vi "Write Sine Grap to binary file.vi"() -> ()   [LabVIEW 2020]
uses:
  <vilib>/Analysis/NI_AALBase.lvlib
panel:
  in  "Path":path
  out "Array":dbl[](array[numeric])
  out "Waveform Graph":dbl[](graph)
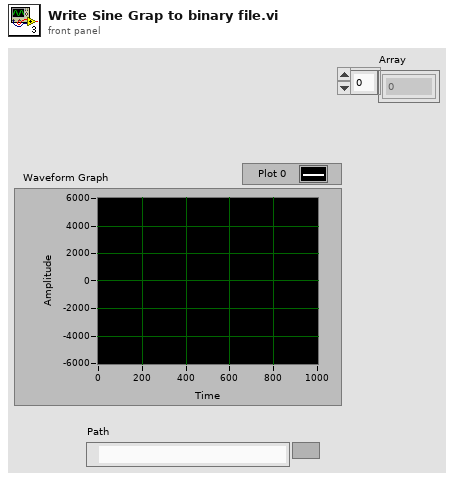
[diagram p1: front panel]
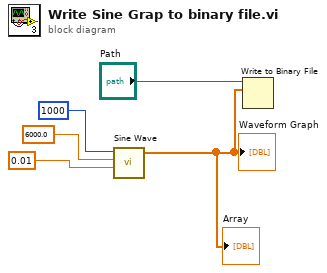
[diagram p0: block diagram]
diagram:
  n1 = call <vilib>:"Sine Wave.vi"("samples"=1000, "amplitude"=6000.0, "frequency"=0.01) -> ("sine wave"=w2:dbl[])  [unwired: 2 in, 2 out]
  "Waveform Graph" <- w2
  "Array" <- w2
  n2 = Write to Binary File(file (use dialog)="Path", data=w2) -> ()  [unwired: 4 in, 3 out]
